vi "Apend Test Case Result to Suite Element.vi"(8 "error in (no error)":errorcluster, 9 "Test Case Result":T1, 10 "Test Suite Element in":refnum<k20>, 11 "XML Report In":refnum<class "XML Report.lvclass">) -> (0 "error out":errorcluster, 2 "Test Suite Element out":refnum<k20>, 3 "XML Report Out":refnum<class "XML Report.lvclass">)   [LabVIEW 2020, in "XML Report.lvclass"]
uses:
  XML Report.lvclass
  Result Types/Case Result/Test Case Result.ctl
  Result Types/Method Result/Method Result.ctl
  Core/Result/Status.ctl
  Result Types/Assertion Result/Assertion Result.ctl
  Result Types/Assertion Result/Public/TypeDefs/Assertion Type.ctl
  Result Types/Assertion Result/Public/TypeDefs/Status.ctl
  XML Report.lvclass/XML Report.ctl
  <vilib>/xml/Close Reference(Node).vi
  <resource>/objmgr/DOMUserDefRef.rc
  Result Types/Case Result/Test Case Result.lvlib
  Result Types/Method Result/Method Result.lvlib
  <vilib>/xml/NI_XML.lvlib
  Result Types/Assertion Result/Assertion Result.lvlib
  Core/Result/Result.lvlib
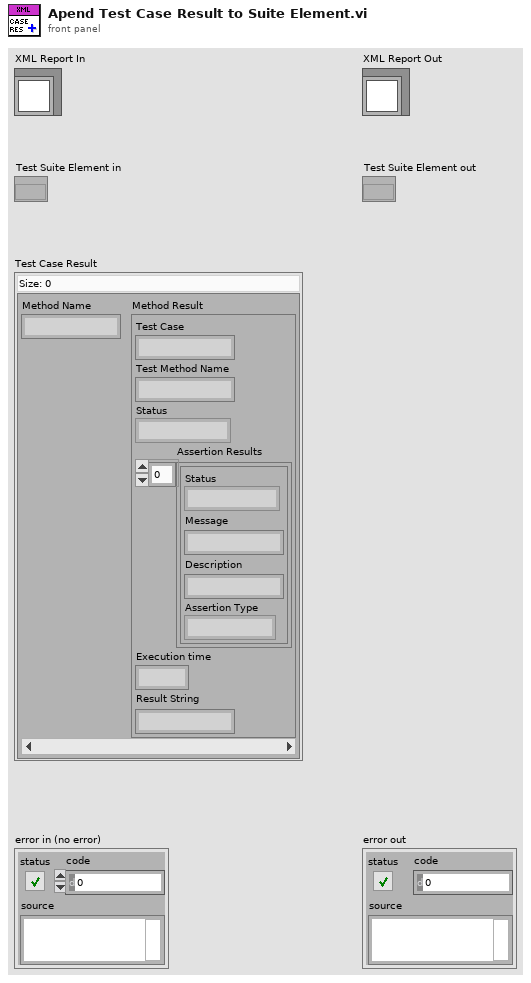
[diagram p1: front panel]
types:
  T1 = typedef "Test Case Result.lvlib/Test Case Result.ctl" = map{string, T2}
  T2 = typedef "Method Result.lvlib/Method Result.ctl" = cluster{"Test Case":string, "Test Method Name":string, "Status":T3, "Assertion Results":T4[], "Execution time":dbl, "Result String":string}
  T3 = typedef "Result.lvlib/Status.ctl" = enum16{"", "Passed", "Failed", "Error", "Skipped", "Setup Error", "Broken", "Teardown Error"}
  T4 = typedef "Assertion Result.lvlib/Assertion Result.ctl" = cluster{"Status":T3, "Message":string, "Description":string, "Assertion Type":T5}
  T5 = typedef "Result.lvlib/Assertion Type.ctl" = enum16{"None", "Pass", "Fail", "Skip", "Pass if Equal", "Fail if Equal", "Pass if Error", "Fail if Error", "Pass if", "Fail if"}
  T6 = typedef "Assertion Result.lvlib/Status.ctl" = enum16{"Pass", "Fail", "Error", "Skipped", "Setup Error", "Broken", "Teardown Error"}
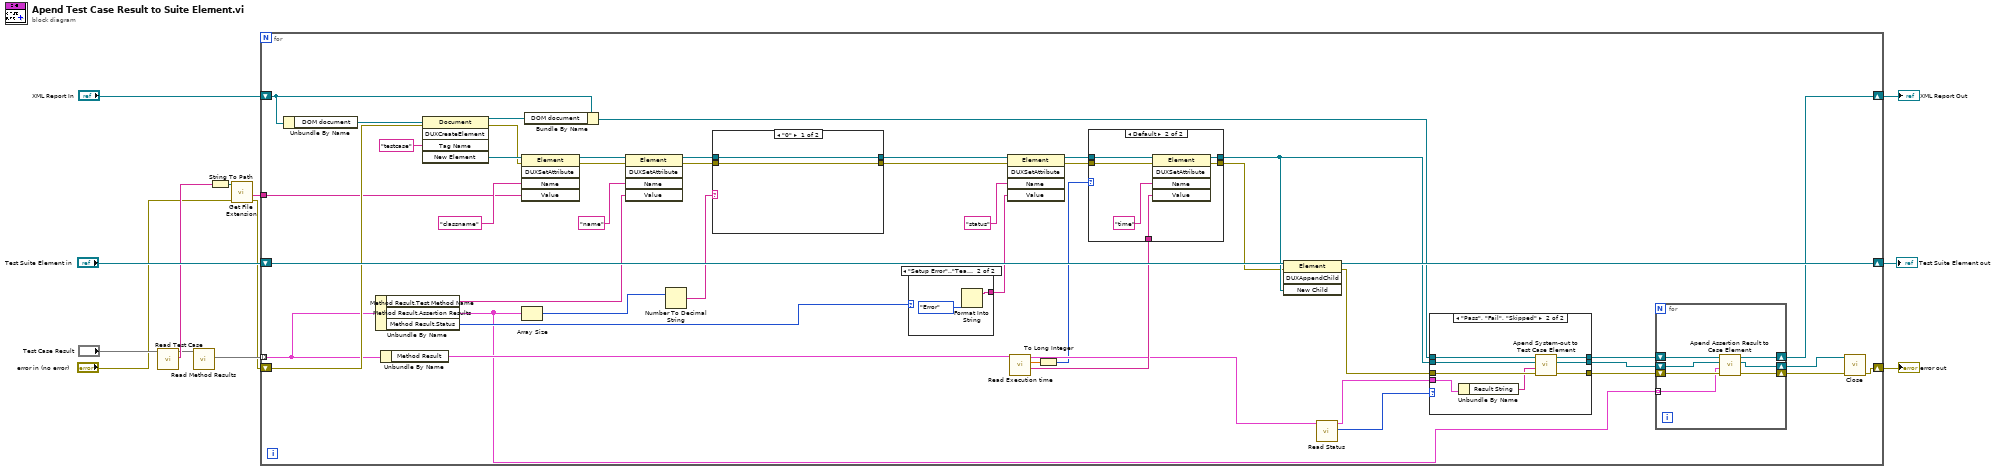
[diagram p0: block diagram]
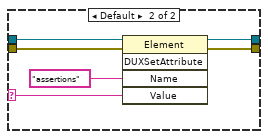
[diagram p3: hidden frame]
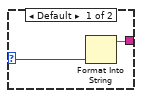
[diagram p4: hidden frame]
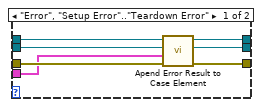
[diagram p5: hidden frame]
diagram:
  n1 = call "Read Test Case.vi"("Test Case Result In"="Test Case Result") -> ("Test Case"=w8:string, "Test Case Result Out"=w7:T1)  [unwired: 9 in]
  n2 = call "Read Method Results.vi"("Test Case Result In"=w7) -> ("Method Results"=w6:map{string, T2})  [unwired: 9 in, 1 out]
  n3 = String To Path(string=w8) -> (path=w4:path)
  n4 = call <vilib>:"Get File Extension.vi"("error in (no error)"="error in (no error)", "file"=w4) -> ("error out"=w2:errorcluster, "filename without extension"=w3:string)  [unwired: 5 in, 3 out]
  n5 = for {
    shift-right: [w59] -> w13
    shift-left: "Test Suite Element in" -> [w57]
    shift-right: [w34] -> w10
    shift-left: "XML Report In" -> [w55]
    tunnel: w6 -> [w20] mode=indexing
    shift-right: [w37] -> w5
    shift-left: w2 -> [w41]
    tunnel: w3 -> [w29]
    n6 = Unbundle By Name(w55) -> ("DOM document"=w56:refnum<k20>)
    n7 = Unbundle By Name(w20) -> ("Method Result.Test Method Name"=w19:string, "Method Result.Assertion Results"=w15:T4[], "Method Result.Status"=w17:T3)
    n8 = Unbundle By Name(w20) -> ("Method Result"=w16:T2)
    n9 = invoke class="Document" method="DUXCreateElement"(reference=w56, error in=w41, "Tag Name"="testcase") -> (reference out=w54:refnum<k20>, error out=w40:errorcluster, "New Element"=w45:refnum<k20>)  [unwired: 2 in, 2 out]
    n10 = invoke class="Element" method="DUXSetAttribute"(reference=w45, error in=w40, "Name"="classname", "Value"=w29) -> (reference out=w53:refnum<k20>, error out=w52:errorcluster)  [unwired: 1 in, 3 out]
    n11 = Array Size(array=w15) -> (size(s)=w21:i32)
    n12 = Bundle By Name(cluster=w55, "DOM document"=w54) -> (w31:refnum<class "XML Report.lvclass">)
    n13 = invoke class="Element" method="DUXSetAttribute"(reference=w53, error in=w52, "Name"="name", "Value"=w19) -> (reference out=w51:refnum<k20>, error out=w50:errorcluster)  [unwired: 1 in, 3 out]
    n14 = Number To Decimal String(number=w21) -> (decimal integer string=w18:string)  [unwired: 1 in]
    n15 = case shown="\"0\"" w18 {
      selector: w18 -> [_ w70]
      tunnel: w51 -> [w69 w75]
      tunnel: w50 -> [w68 w74]
      tunnel: [w69 w73] -> w49
      tunnel: [w68 w72] -> w48
      frame "0" {
      }
      frame Default {
        n16 = invoke class="Element" method="DUXSetAttribute"(reference=w75, error in=w74, "Name"="assertions", "Value"=w70) -> (reference out=w73:refnum<k20>, error out=w72:errorcluster)  [unwired: 1 in, 3 out]
      }
    }
    n17 = case shown="\"Setup Error\"..\"Teardown Error\"" w17 {
      selector: w17 -> [w76 _]
      tunnel: [w77 w78] -> w39
      frame Default {
        n18 = Format Into String(w76) -> (resulting string=w77:string)  [unwired: 3 in, 1 out]
      }
      frame "Setup Error".."Teardown Error" {
        n19 = Format Into String(Status."Error" ("Status")) -> (resulting string=w78:string)  [unwired: 3 in, 1 out]
      }
    }
    n20 = invoke class="Element" method="DUXSetAttribute"(reference=w49, error in=w48, "Name"="status", "Value"=w39) -> (reference out=w47:refnum<k20>, error out=w46:errorcluster)  [unwired: 1 in, 3 out]
    n21 = call "Read Execution time.vi"("Method Result In"=w16) -> ("Execution time string"=w38:string, "Execution time"=w28:dbl, "Method Result Out"=w33:T2)  [unwired: 8 in]
    n22 = To Long Integer(number=w28) -> (32bit integer=w27:i32)
    n23 = case shown="Default" w27 {
      tunnel: w47 -> [w60 w67]
      tunnel: w46 -> [w61 w66]
      tunnel: w38 -> [_ w64]
      tunnel: [w60 w63] -> w32
      tunnel: [w61 w62] -> w30
      frame 0 {
      }
      frame Default {
        n24 = invoke class="Element" method="DUXSetAttribute"(reference=w67, error in=w66, "Name"="time", "Value"=w64) -> (reference out=w63:refnum<k20>, error out=w62:errorcluster)  [unwired: 1 in, 3 out]
      }
    }
    n25 = invoke class="Element" method="DUXAppendChild"(reference=w57, error in=w30, "New Child"=w32) -> (reference out=w59:refnum<k20>, error out=w23:errorcluster)  [unwired: 1 in, 2 out]
    n26 = call "Read Status.vi"("Method Result In"=w33) -> ("Status"=w26:T6, "Method Result Out"=w14:T2)  [unwired: 8 in, 1 out]
    n27 = case shown="\"Pass\", \"Fail\", \"Skipped\"" w26 {
      tunnel: w31 -> [w93 w100]
      tunnel: [w92 w99] -> w25
      tunnel: [w91 w98] -> w24
      tunnel: w32 -> [w90 w95]
      tunnel: w23 -> [w89 w96]
      tunnel: [w88 w97] -> w22
      tunnel: w14 -> [w87 w101]
      frame "Error", "Setup Error".."Teardown Error" {
        n28 = call "Apend Error Result to Case Element.vi"("error in (no error)"=w89, "Method Result"=w87, "Test Case Element in"=w90, "XML Report In"=w93) -> ("error out"=w88:errorcluster, "Test Case Element out"=w91:refnum<k20>, "XML Report Out"=w92:refnum<class "XML Report.lvclass">)  [unwired: 5 in]
      }
      frame "Pass", "Fail", "Skipped" {
        n29 = Unbundle By Name(w101) -> ("Result String"=w94:string)
        n30 = call "Apend System-out to Test Case Element.vi"("error in (no error)"=w96, "Result String"=w94, "Test Case Element in"=w95, "XML Report In"=w100) -> ("error out"=w97:errorcluster, "Test Case Element out"=w98:refnum<k20>, "XML Report Out"=w99:refnum<class "XML Report.lvclass">)  [unwired: 5 in]
      }
    }
    n31 = for {
      shift-right: [w85] -> w36
      shift-left: w24 -> [w86]
      shift-right: [w82] -> w34
      shift-left: w25 -> [w83]
      shift-right: [w84] -> w35
      shift-left: w22 -> [w81]
      tunnel: w15 -> [w80] mode=indexing
      n32 = call "Apend Assertion Result to Case Element.vi"("error in (no error)"=w81, "Assertion Result"=w80, "Test Case Element in"=w86, "XML Report In"=w83) -> ("error out"=w84:errorcluster, "Test Case Element out"=w85:refnum<k20>, "XML Report Out"=w82:refnum<class "XML Report.lvclass">)  [unwired: 5 in]
    }
    n33 = call-poly <vilib>:"Close.vi"("error in (no error)"=w35, "node"=w36) -> ("error out"=w37:errorcluster)  [unwired: 7 in]
  }
  "error out" <- w5
  "Test Suite Element out" <- w13
  "XML Report Out" <- w10
